vi "ordenado.vi"() -> ()   [LabVIEW 2013]
uses:
  <vilib>/LabVIEW Interface for Arduino/LabVIEW Interface for Arduino.lvlib
panel:
  out "LSB":dbl
  out "MSB":dbl
  out "I2C Data":u8[](array[numeric])
  in  "stop":bool
  out "Accion":string
  in  "Consigna":dbl(knob) scale=0.0..360.0
  out "CASE":dbl
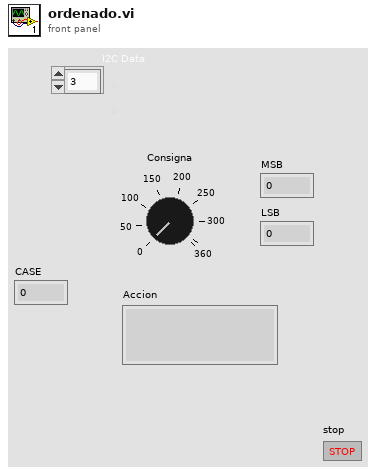
[diagram p1: front panel]
types:
  T1 = typedef "LabVIEW Interface for Arduino.lvlib/Arduino Resource.ctl" = cluster{"VISA resource":refnum<visa-resource-name>, "Board Type":T2, "Connection Type":enum8{"USB / Serial"}, "Bytes Per Packet (15)":u8}
  T2 = typedef "LabVIEW Interface for Arduino.lvlib/Board Type.ctl" = enum16{"Uno", "Dimuelanove w/Atmega 328", "Mega 2560"}
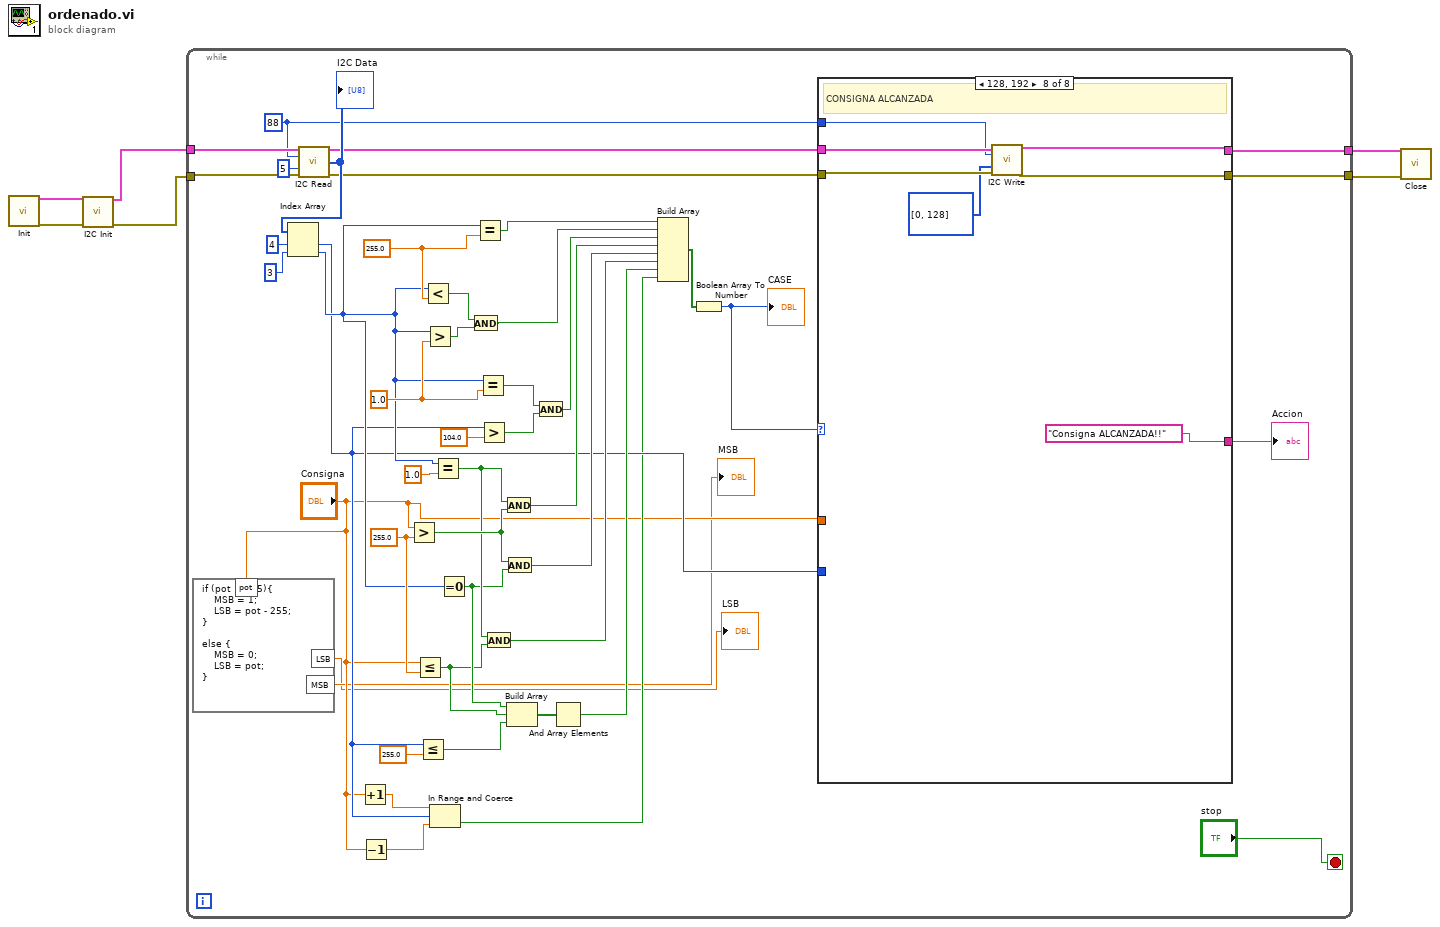
[diagram p0: block diagram]
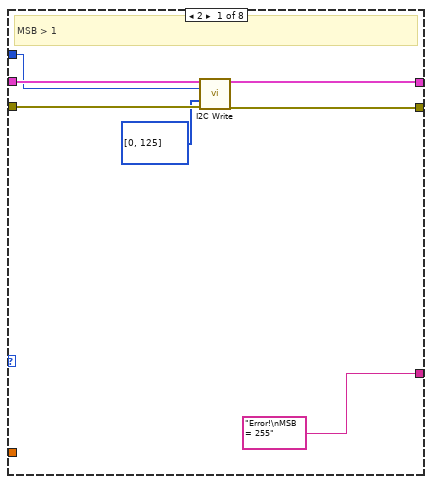
[diagram p2: hidden frame]
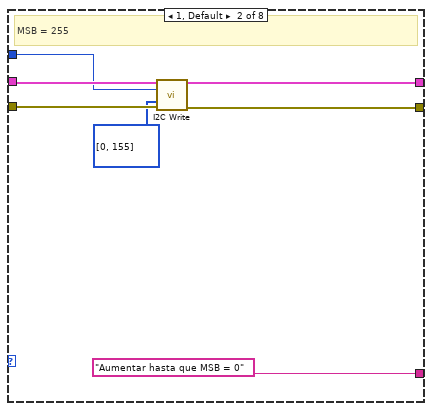
[diagram p3: hidden frame]
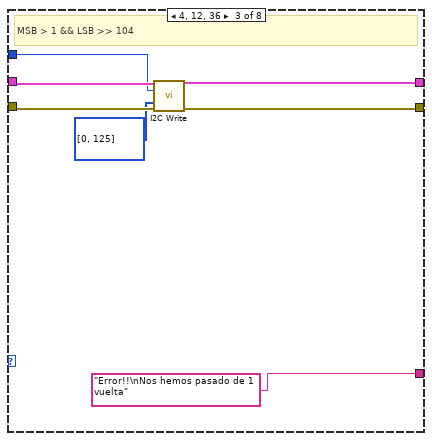
[diagram p4: hidden frame]
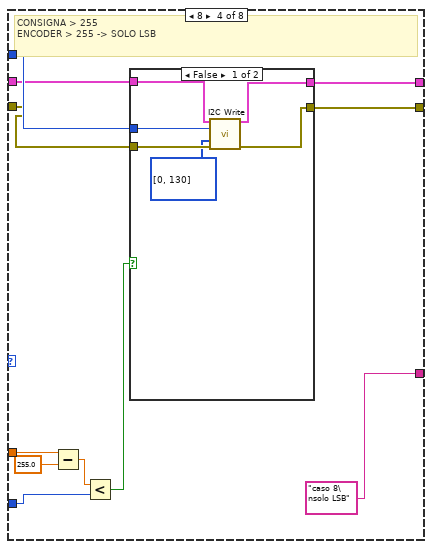
[diagram p5: hidden frame]
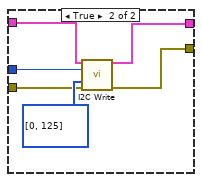
[diagram p6: hidden frame]
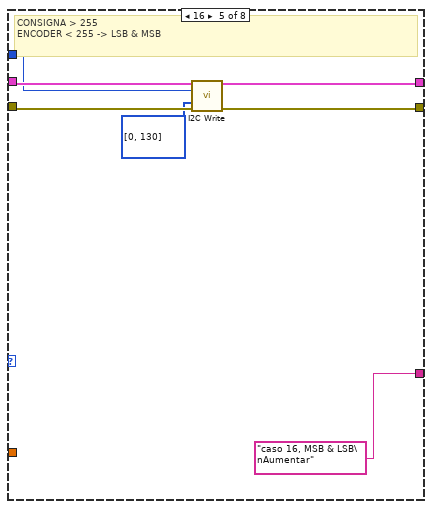
[diagram p7: hidden frame]
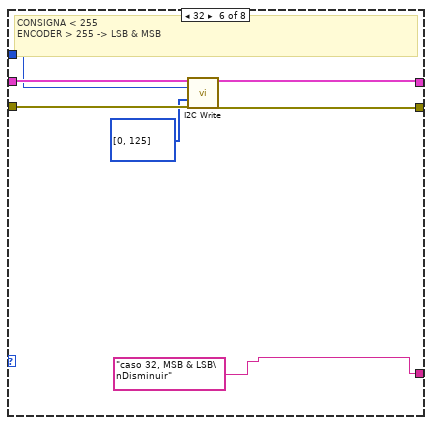
[diagram p8: hidden frame]
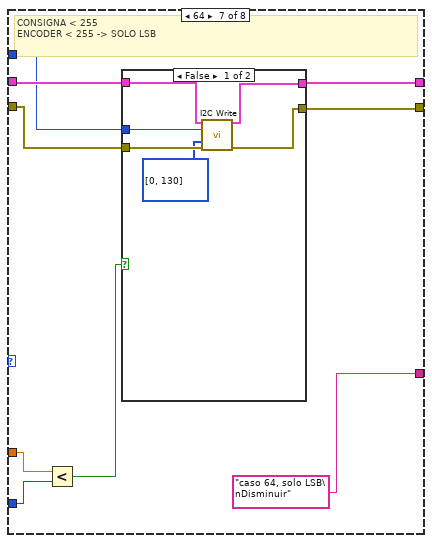
[diagram p9: hidden frame]
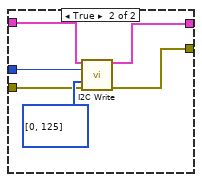
[diagram p10: hidden frame]
diagram:
  n1 = call <vilib>:"Init.vi"() -> ("Arduino Resource"=w6:T1, "error out"=w5:errorcluster)  [unwired: 18 in]
  n2 = call <vilib>:"I2C Init.vi"("Arduino Resource"=w6, "error in"=w5) -> ("Arduino Resource"=w4:T1, "error out"=w3:errorcluster)  [unwired: 12 in]
  n3 = while {
    tunnel: w4 -> [w25]
    tunnel: w3 -> [w24]
    tunnel: [w16] -> w2
    tunnel: [w15] -> w1
    stop <- "stop" stop-if-true
    w14 = u8 88 ("Address (0)")
    w42 = 255.0 ("y")
    w32 = 1.0 ("y")
    w33 = 255.0 ("y")
    n4 = formula code="if (pot > 255){\n    MSB = 1;\n    LSB = pot - 255;\n}\n\nelse {\n    MSB = 0;\n    LSB = pot;\n}"("pot"="Consigna") -> ("MSB"=→"MSB":dbl, "LSB"=→"LSB":dbl)
    n5 = call <vilib>:"I2C Read.vi"("Arduino Resource"=w25, "Address (0)"=w14, "Bytes To Read"=u8 5, "error in"=w24) -> ("Arduino Resource"=w18:T1, "I2C Data"=w22:u8[], "error out"=w17:errorcluster)  [unwired: 9 in]
    "I2C Data" <- w22
    n6 = Index Array(array=w22, index #1=4 ("index"), index #2=3 ("index")) -> (element #1=w13:u8, element #2=w19:u8)
    n7 = Increment(x="Consigna") -> (x+1=w12:dbl)
    n8 = Decrement(x="Consigna") -> (x-1=w11:dbl)
    n9 = Greater?(x="Consigna", y=w42) -> (0:w44:bool)
    n10 = Less Or Equal?(x="Consigna", y=w42) -> (x <= y?=w37:bool)
    n11 = Less Or Equal?(x=w13, y=255.0) -> (x <= y?=w36:bool)
    n12 = Less?(x=w19, y=w33) -> (x < y?=w30:bool)
    n13 = Greater?(x=w19, y=w32) -> (0:w31:bool)
    n14 = In Range and Coerce(upper limit=w12, x=w13, lower limit=w11) -> (In Range?=w10:bool)  [unwired: 1 out]
    n15 = Equal?(x=w19, y=1.0) -> (x = y?=w41:bool)
    n16 = Equal To 0?(x=w19) -> (x = 0?=w38:bool)
    n17 = And(x=w30, y=w31) -> (x .and. y?=w29:bool)
    n18 = Equal?(x=w19, y=w33) -> (x = y?=w52:bool)
    n19 = Equal?(x=w19, y=w32) -> (x = y?=w51:bool)
    n20 = Greater?(x=w13, y=104.0) -> (0:w50:bool)
    n21 = And(x=w41, y=w37) -> (x .and. y?=w40:bool)
    n22 = And(x=w41, y=w44) -> (x .and. y?=w45:bool)
    n23 = And(x=w44, y=w38) -> (x .and. y?=w43:bool)
    n24 = Build Array(w38, w37, w36) -> (w35:bool[])
    n25 = And(x=w51, y=w50) -> (x .and. y?=w49:bool)
    n26 = And Array Elements(Boolean array=w35) -> (logical AND=w34:bool)
    n27 = Build Array(w52, w29, w49, w45, w43, w40, w34, w10) -> (w48:bool[])
    n28 = Boolean Array To Number(Boolean array=w48) -> (number=w28:u32)
    "CASE" <- w28
    n29 = case shown="128, 192" w28 {
      tunnel: ["Error!\nMSB = 255" "Aumentar hasta que MSB = 0" "Error!!\nNos hemos pasado de 1 vuelta" "caso 8\nsolo LSB" "caso 16, MSB & LSB\nAumentar" "caso 32, MSB & LSB\nDisminuir" "caso 64, solo LSB\nDisminuir" "Consigna ALCANZADA!!"] -> w27
      tunnel: w18 -> [w55 w65 w72 w77 w99 w109 w118 w138]
      tunnel: w17 -> [w56 w64 w71 w76 w100 w108 w116 w137]
      tunnel: [w58 w63 w69 w74 w102 w107 w114 w136] -> w16
      tunnel: [w57 w62 w70 w75 w101 w106 w115 w135] -> w15
      tunnel: w14 -> [w54 w61 w68 w78 w98 w105 w117 w134]
      tunnel: "Consigna" -> [_ _ _ w83 _ _ w113 _]
      tunnel: w13 -> [_ _ _ w80 _ _ w112 _]
      frame 2 {
        # "MSB > 1"
        n30 = call <vilib>:"I2C Write.vi"("Arduino Resource"=w55, "Address (0)"=w54, "I2C Data Bytes"=u8[] [0, 125], "error in"=w56) -> ("Arduino Resource"=w58:T1, "error out"=w57:errorcluster)  [unwired: 10 in]
      }
      frame 1, Default {
        # "MSB = 255"
        n31 = call <vilib>:"I2C Write.vi"("Arduino Resource"=w65, "Address (0)"=w61, "I2C Data Bytes"=u8[] [0, 155], "error in"=w64) -> ("Arduino Resource"=w63:T1, "error out"=w62:errorcluster)  [unwired: 10 in]
      }
      frame 4, 12, 36 {
        # "MSB > 1 && LSB >> 104"
        n32 = call <vilib>:"I2C Write.vi"("Arduino Resource"=w72, "Address (0)"=w68, "I2C Data Bytes"=u8[] [0, 125], "error in"=w71) -> ("Arduino Resource"=w69:T1, "error out"=w70:errorcluster)  [unwired: 10 in]
      }
      frame 8 {
        # "CONSIGNA > 255\nENCODER > 255 -> SOLO LSB"
        n33 = Subtract(x=w83, y=255.0) -> (x-y=w81:dbl)
        n34 = Less?(x=w81, y=w80) -> (x < y?=w79:bool)
        n35 = case shown="False" w79 {
          tunnel: w78 -> [w89 w95]
          tunnel: w77 -> [w90 w94]
          tunnel: w76 -> [w88 w93]
          tunnel: [w86 w92] -> w75
          tunnel: [w87 w91] -> w74
          frame False {
            n36 = call <vilib>:"I2C Write.vi"("Arduino Resource"=w90, "Address (0)"=w89, "I2C Data Bytes"=u8[] [0, 130], "error in"=w88) -> ("Arduino Resource"=w87:T1, "error out"=w86:errorcluster)  [unwired: 10 in]
          }
          frame True {
            n37 = call <vilib>:"I2C Write.vi"("Arduino Resource"=w94, "Address (0)"=w95, "I2C Data Bytes"=u8[] [0, 125], "error in"=w93) -> ("Arduino Resource"=w91:T1, "error out"=w92:errorcluster)  [unwired: 10 in]
          }
        }
      }
      frame 16 {
        # "CONSIGNA > 255\nENCODER < 255 -> LSB & MSB"
        n38 = call <vilib>:"I2C Write.vi"("Arduino Resource"=w99, "Address (0)"=w98, "I2C Data Bytes"=u8[] [0, 130], "error in"=w100) -> ("Arduino Resource"=w102:T1, "error out"=w101:errorcluster)  [unwired: 10 in]
      }
      frame 32 {
        # "CONSIGNA < 255\nENCODER > 255 -> LSB & MSB"
        n39 = call <vilib>:"I2C Write.vi"("Arduino Resource"=w109, "Address (0)"=w105, "I2C Data Bytes"=u8[] [0, 125], "error in"=w108) -> ("Arduino Resource"=w107:T1, "error out"=w106:errorcluster)  [unwired: 10 in]
      }
      frame 64 {
        # "CONSIGNA < 255\nENCODER < 255 -> SOLO LSB"
        n40 = Less?(x=w113, y=w112) -> (x < y?=w111:bool)
        n41 = case shown="False" w111 {
          tunnel: w117 -> [w124 w130]
          tunnel: w118 -> [w125 w129]
          tunnel: w116 -> [w123 w128]
          tunnel: [w121 w127] -> w115
          tunnel: [w122 w126] -> w114
          frame False {
            n42 = call <vilib>:"I2C Write.vi"("Arduino Resource"=w125, "Address (0)"=w124, "I2C Data Bytes"=u8[] [0, 130], "error in"=w123) -> ("Arduino Resource"=w122:T1, "error out"=w121:errorcluster)  [unwired: 10 in]
          }
          frame True {
            n43 = call <vilib>:"I2C Write.vi"("Arduino Resource"=w129, "Address (0)"=w130, "I2C Data Bytes"=u8[] [0, 125], "error in"=w128) -> ("Arduino Resource"=w126:T1, "error out"=w127:errorcluster)  [unwired: 10 in]
          }
        }
      }
      frame 128, 192 {
        # "CONSIGNA ALCANZADA"
        n44 = call <vilib>:"I2C Write.vi"("Arduino Resource"=w138, "Address (0)"=w134, "I2C Data Bytes"=u8[] [0, 128], "error in"=w137) -> ("Arduino Resource"=w136:T1, "error out"=w135:errorcluster)  [unwired: 10 in]
      }
    }
    "Accion" <- w27
  }
  n45 = call <vilib>:"Close.vi"("Arduino Resource"=w2, "error in"=w1) -> ()  [unwired: 13 in, 1 out]
